vi "Averaged Power Spectrum.vi"(0 "scaled signal [EU]":dbl[](array[numeric]) format="%.2f", 1 "sampling frequency [Hz]":dbl=10000.0 format="%.2f", 2 "window":T6 items=["Rectangle"=0, "Hanning"=1, "Hamming"=2, "Blackman-Harris"=3, "Exact Blackman"=4, "Blackman"=5, "Flat Top"=6, "4 Term B-Harris "=7, "7 Term B-Harris"=8, "Low Sidelobe"=9, "Blackman Nuttall"=11, "Triangle"=30, "Bartlett-Hanning"=31, "Bohman"=32, "Parzen"=33, "Welch"=34, "Kaiser"=60, "Dolph-Chebyshev"=61, "Gaussian"=62], 4 "dB On (F)":bool, 5 "channel info":T1={"sensor sensitivity [mV/EU]"=1000.0, "engineering units"=1, "dB reference [EU]"=1.0, "custom label"="EU", "weighting filter"=0, "pregain [dB]"=0.0} {"pregain [dB]" format="%.2f"; "weighting filter" items=["Linear", "A-weighting", "B-weighting", "C-weighting", "ITU-R 468-4", "Dolby", "CCITT", "C-message"]; "dB reference [EU]" format="%^.1e"; "engineering units" items=["custom..."=0, "V"=1, "A"=21, "Pa"=2, "N"=20, "g"=3, "m/s^2"=4, "m/s"=5, "m"=6, "mm/s"=12, "mm"=13, "microns/s"=14, "microns"=15, "in/s^2"=7, "in/s"=8, "in"=9, "mils/s"=10, "mils"=11, "rad/s^2"=16, "rad/s"=17, "rad"=18, "strain"=19]; "sensor sensitivity [mV/EU]" format="%.2f"}, 6 "frequency weighting":T5(ring), 7 "reset averaging (T)":bool=TRUE, 9 "averaging parameters":T4={"averaging mode"=enum."RMS averaging", "weighting mode"=enum."Linear", "number of averages"=10} {"number of averages" min=1}) -> (11 "window constants":cluster{"eq noise BW":dbl, "coherent gain":dbl} {"coherent gain" format="%.2f"; "eq noise BW" format="%.2f"}, 13 "weighting conflict":bool, 14 "power spectrum [EU^2 rms]":dbl[](array[numeric]) format="%.2f", 15 "unit label":string, 16 "df [Hz]":dbl format="%.2f", 18 "averages completed":dbl format="%.2f", 19 "error out":errorcluster)   [LabVIEW 2017]
doc: "Computes the averaged power spectrum of the input signal.\nEach block of data corresponds to a single FFT block and has to be passed individually to this VI. The first time this VI is called, reset averaging must be TRUE (default value), to start a new averaging process. For subsequent calls, reset averaging must be FALSE to continue the averaging process. Averages completed returns the number of averages completed so far.\nAveraging parameters specifies how the averaging is performed. This includes the averaging mode (no averaging, vector averaging, RMS averaging, or peak hold), the weighting mode (linear or exponential), and the number of averages (used only if the weighting mode is exponential).\nThe selected frequency weighting (A, B, or C) is applied to the results in the frequency domain (no time-domain filtering operation)."
uses:
  <vilib>/Analysis/4window.llb/windowTd.ctl
  <vilib>/addons/Sound and Vibration/compatibility/Controls/svl_Channel Info.ctl
  <vilib>/addons/Sound and Vibration/compatibility/Controls/svl_Engineering Units Text Ring.ctl
  <vilib>/addons/Sound and Vibration/compatibility/Controls/svl_Weighting Filter Text Ring.ctl
  <vilib>/Analysis/2dsp.llb/Power Spectrum (DBL).vi
  <vilib>/Analysis/2dsp.llb/Real FFT.vi
  <vilib>/Analysis/0measdsp.llb/Scaled Time Domain Window (DBL).vi
  <vilib>/Analysis/NI_AALPro.lvlib
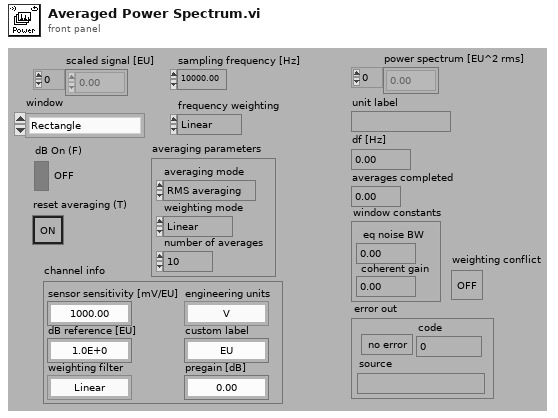
[diagram p1: front panel]
types:
  T1 = typedef "svl_Channel Info.ctl" = cluster{"sensor sensitivity [mV/EU]":dbl, "engineering units":T2, "dB reference [EU]":dbl, "custom label":string, "weighting filter":T3, "pregain [dB]":dbl}
  T2 = typedef "svl_Engineering Units Text Ring.ctl" = u16
  T3 = typedef "svl_Weighting Filter Text Ring.ctl" = u16
  T4 = cluster{"averaging mode":enum16{"No averaging", "Vector averaging", "RMS averaging", "Peak hold"}, "weighting mode":enum16{"Linear", "Exponential"}, "number of averages":u32}
  T5 = enum16{"Linear", "A-weighting", "B-weighting", "C-weighting"}
  T6 = typedef "NI_AALPro.lvlib/windowTd.ctl" = u32
  T7 = enum16{"No averaging", "Vector averaging", "RMS averaging", "Peak hold"}
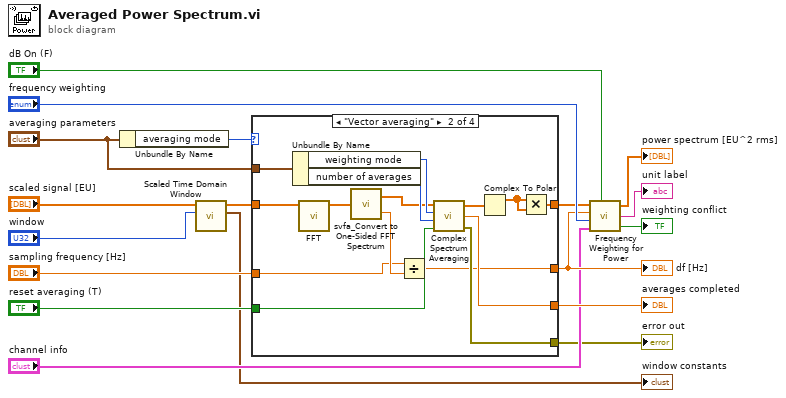
[diagram p0: block diagram]
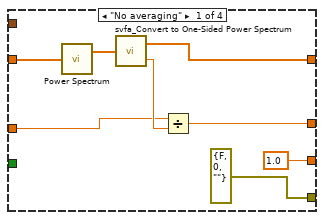
[diagram p2: hidden frame]
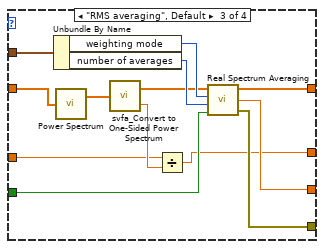
[diagram p3: hidden frame]
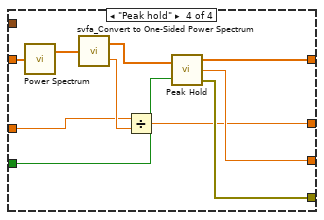
[diagram p4: hidden frame]
diagram:
  n1 = Unbundle By Name("averaging parameters") -> ("averaging mode"=w9:T7)
  n2 = call-poly <vilib>:"Scaled Time Domain Window.vi"("window"="window", "X"="scaled signal [EU]") -> ("window properties"=→"window constants":cluster{"eq noise BW":dbl, "coherent gain":dbl}, "Windowed X"=w13:dbl[])  [unwired: 7 in, 1 out]
  n3 = case shown="\"Vector averaging\"" w9 {
    tunnel: w13 -> [w22 w31 w45 w58]
    tunnel: "sampling frequency [Hz]" -> [w19 w27 w43 w56]
    tunnel: [w20 w28 w42 w55] -> w11
    tunnel: [w21 w37 w52 w62] -> w10
    tunnel: "averaging parameters" -> [_ w41 w54 _]
    tunnel: "reset averaging (T)" -> [_ w40 w53 w64]
    tunnel: [1.0 ("averages completed") w36 w51 w63] -> w6
    tunnel: [errorcluster {"status"=FALSE, "code"=0, "source"=""} ("error out") w35 w50 w61] -> w2
    frame "No averaging" {
      n4 = call-poly <vilib>:"Power Spectrum.vi"("X"=w22) -> ("Power Spectrum"=w23:dbl[])  [unwired: 1 out]
      n5 = call <vilib>:"svfa_Convert to One-Sided Power Spectrum.vi"("two-sided power spectrum"=w23) -> ("one-sided power spectrum"=w21:dbl[], "block size"=w24:dbl)
      n6 = Divide(x=w19, y=w24) -> (x/y=w20:dbl)
    }
    frame "Vector averaging" {
      n7 = Unbundle By Name(w41) -> ("weighting mode"=w34:enum16{"Linear", "Exponential"}, "number of averages"=w33:u32)
      n8 = call-poly <vilib>:"FFT.vi"("X"=w31) -> ("FFT {X}"=w30:cdb[])  [unwired: 9 in, 1 out]
      n9 = call <vilib>:"svfa_Convert to One-Sided FFT Spectrum.vi"("two-sided FFT spectrum"=w30) -> ("one-sided FFT spectrum"=w29:cdb[], "block size"=w32:dbl)
      n10 = Divide(x=w27, y=w32) -> (x/y=w28:dbl)
      n11 = call <vilib>:"Complex Spectrum Averaging.vi"("reset averaging (T)"=w40, "number of averages"=w33, "weighting mode"=w34, "complex spectrum"=w29) -> ("error out"=w35:errorcluster, "averages completed"=w36:dbl, "averaged complex spectrum"=w39:cdb[])
      n12 = Complex To Polar(r * e^(i*theta)=w39) -> (r=w38:dbl[])  [unwired: 1 out]
      n13 = Multiply(x=w38, y=w38) -> (x*y=w37:dbl[])
    }
    frame "RMS averaging", Default {
      n14 = Unbundle By Name(w54) -> ("weighting mode"=w49:enum16{"Linear", "Exponential"}, "number of averages"=w48:u32)
      n15 = call-poly <vilib>:"Power Spectrum.vi"("X"=w45) -> ("Power Spectrum"=w46:dbl[])  [unwired: 1 out]
      n16 = call <vilib>:"svfa_Convert to One-Sided Power Spectrum.vi"("two-sided power spectrum"=w46) -> ("one-sided power spectrum"=w44:dbl[], "block size"=w47:dbl)
      n17 = Divide(x=w43, y=w47) -> (x/y=w42:dbl)
      n18 = call <vilib>:"Real Spectrum Averaging.vi"("reset averaging (T)"=w53, "number of averages"=w48, "weighting mode"=w49, "real spectrum"=w44) -> ("error out"=w50:errorcluster, "averages completed"=w51:dbl, "averaged real spectrum"=w52:dbl[])
    }
    frame "Peak hold" {
      n19 = call-poly <vilib>:"Power Spectrum.vi"("X"=w58) -> ("Power Spectrum"=w59:dbl[])  [unwired: 1 out]
      n20 = call <vilib>:"svfa_Convert to One-Sided Power Spectrum.vi"("two-sided power spectrum"=w59) -> ("one-sided power spectrum"=w57:dbl[], "block size"=w60:dbl)
      n21 = Divide(x=w56, y=w60) -> (x/y=w55:dbl)
      n22 = call <vilib>:"Peak Hold.vi"("real spectrum"=w57, "reset averaging"=w64) -> ("peak spectrum"=w62:dbl[], "averages completed"=w63:dbl, "error out"=w61:errorcluster)
    }
  }
  "df [Hz]" <- w11
  "averages completed" <- w6
  "error out" <- w2
  n23 = call <vilib>:"Frequency Weighting for Power.vi"("power spectrum [EUrms^2]"=w10, "df [Hz]"=w11, "frequency weighting"="frequency weighting", "channel info"="channel info", "dB On (F)"="dB On (F)") -> ("frequency weighted power [EUrms^2]"=→"power spectrum [EU^2 rms]":dbl[], "unit label"=→"unit label":string, "weighting conflict"=→"weighting conflict":bool)
